vi "S2DS_CheckingScanOverInX.vi"(1 "Scan parameters in (old)":T1 {"Y data taking" items=["in both direction", "in up direction only", "in down direction only"]; "X data taking" items=["in both direction", "in up direction only", "in down direction only"]}, 2 "Scan parameters in (new)":T1 {"Y data taking" items=["in both direction", "in up direction only", "in down direction only"]; "X data taking" items=["in both direction", "in up direction only", "in down direction only"]}) -> (0 "Scan parameters out":T1 {"Y data taking" items=["in both direction", "in up direction only", "in down direction only"]; "X data taking" items=["in both direction", "in up direction only", "in down direction only"]})   [LabVIEW 2025]
uses:
  TYPE DEFS/S2DS_Sweep Info.ctl
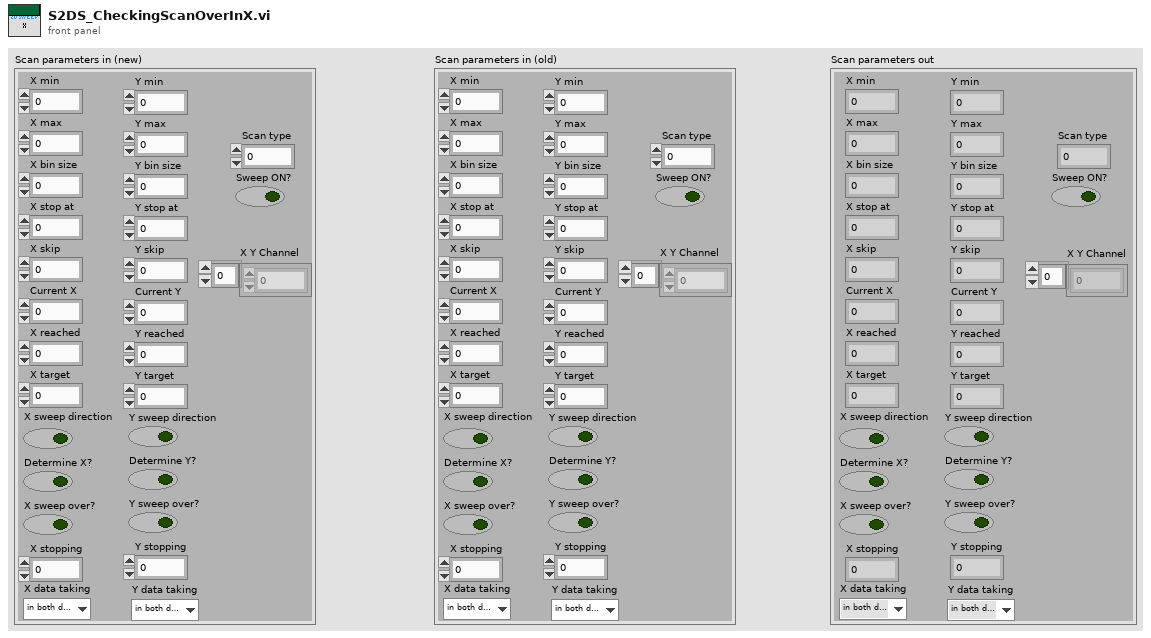
[diagram p1: front panel]
types:
  T1 = typedef "S2DS_Sweep Info.ctl" = cluster{"X min":ext, "X max":dbl, "Y min":dbl, "Y max":dbl, "X bin size":dbl, "Y bin size":dbl, "X stop at":dbl, "Y stop at":dbl, "X skip":u64, "Y skip":u64, "Current X":dbl, "Current Y":dbl, "X reached":i32, "Y reached":i32, "X target":dbl, "Y target":dbl, "Sweep ON?":bool, "X sweep direction":bool, "Y sweep direction":bool, "Determine X?":bool, "Determine Y?":bool, "X sweep over?":bool, "Y sweep over?":bool, "Scan type":i32, "X stopping":i32, "Y stopping":i32, "X Y Channel":u16[], "X data taking":u16, "Y data taking":u16}
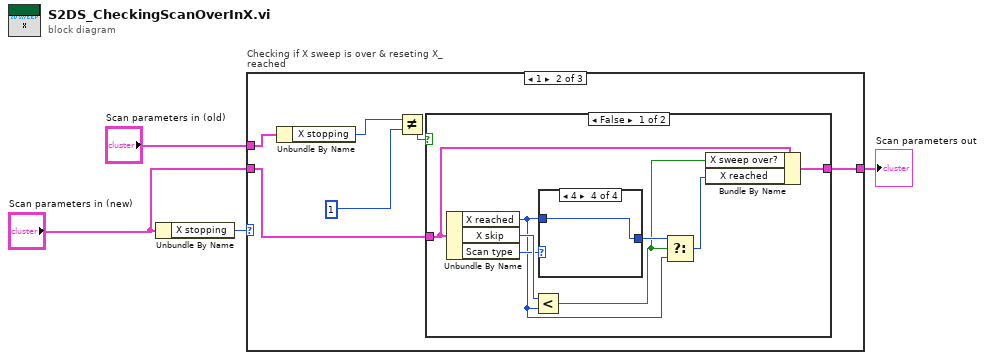
[diagram p0: block diagram]
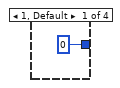
[diagram p3: hidden frame]
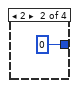
[diagram p4: hidden frame]
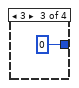
[diagram p5: hidden frame]
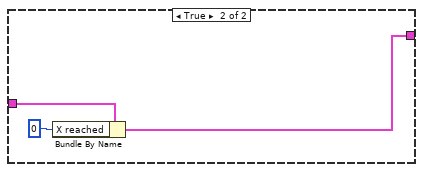
[diagram p6: hidden frame]
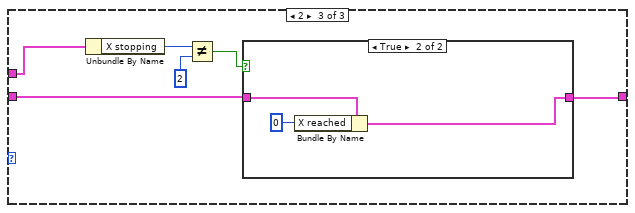
[diagram p7: hidden frame]
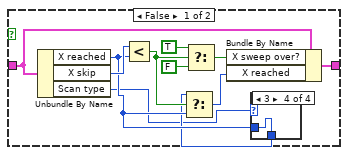
[diagram p8: hidden frame]
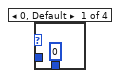
[diagram p9: hidden frame]
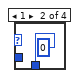
[diagram p10: hidden frame]
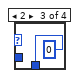
[diagram p11: hidden frame]
diagram:
  n1 = Unbundle By Name("Scan parameters in (new)") -> ("X stopping"=w4:i32)
  n2 = case "Checking if X sweep is over & reseting X_reached" shown="1" w4 {
    tunnel: "Scan parameters in (old)" -> [_ w11 w29]
    tunnel: "Scan parameters in (new)" -> [w5 w7 w28]
    tunnel: [w5 w9 w27] -> w1
    frame 0, Default {
    }
    frame 1 {
      n3 = Unbundle By Name(w11) -> ("X stopping"=w10:i32)
      n4 = Not Equal?(x=w10, y=1) -> (x != y?=w8:bool)
      n5 = case shown="False" w8 {
        tunnel: w7 -> [w19 w25]
        tunnel: [w18 w24] -> w9
        frame False {
          n6 = Unbundle By Name(w19) -> ("X reached"=w14:i32, "X skip"=w17:u64, "Scan type"=w15:i32)
          n7 = Less?(x=w17, y=w14) -> (x < y?=w12:bool)
          n8 = case shown="4" w15 {
            tunnel: [0 0 0 w23] -> w13
            tunnel: w14 -> [_ _ _ w23]
            frame 1, Default {
            }
            frame 2 {
            }
            frame 3 {
            }
            frame 4 {
            }
          }
          n9 = Select(t=w13, s=w12, f=w14) -> (s? t:f=w16:i32)
          n10 = Bundle By Name(cluster=w19, "X sweep over?"=w12, "X reached"=w16) -> (w18:T1)
        }
        frame True {
          n11 = Bundle By Name(cluster=w25, "X reached"=0) -> (w24:T1)
        }
      }
    }
    frame 2 {
      n12 = Unbundle By Name(w29) -> ("X stopping"=w32:i32)
      n13 = Not Equal?(x=w32, y=2) -> (x != y?=w30:bool)
      n14 = case shown="True" w30 {
        tunnel: w28 -> [w40 w49]
        tunnel: [w39 w48] -> w27
        frame False {
          n15 = Unbundle By Name(w40) -> ("X reached"=w35:i32, "X skip"=w37:u64, "Scan type"=w33:i32)
          n16 = Less?(x=w37, y=w35) -> (x < y?=w38:bool)
          n17 = Select(t=TRUE, s=w38, f=FALSE) -> (s? t:f=w41:bool)
          n18 = case shown="3" w33 {
            tunnel: [0 0 0 w47] -> w34
            tunnel: w35 -> [_ _ _ w47]
            frame 0, Default {
            }
            frame 1 {
            }
            frame 2 {
            }
            frame 3 {
            }
          }
          n19 = Select(t=w34, s=w38, f=w35) -> (s? t:f=w36:i32)
          n20 = Bundle By Name(cluster=w40, "X sweep over?"=w41, "X reached"=w36) -> (w39:T1)
        }
        frame True {
          n21 = Bundle By Name(cluster=w49, "X reached"=0) -> (w48:T1)
        }
      }
    }
  }
  "Scan parameters out" <- w1
